vi "FilterSelectionParamSetting.vi"(8 "Error In":errorcluster, 10 "FiltersParam":T1={"Kernel"=[[1.0, 1.0, 1.0], [1.0, 1.0, 1.0], [1.0, 1.0, 1.0]], "Kernel Size"=0, "Filter Size X"=0, "Filter Size Y"=0, "Tolerance %"=0, "Divider"=0.0, "FilterFunction"=enum."Smoothing - Low Pass", "Sigma"=0.0, "LThres"=0.0, "HThresh"=0.0, "Windows Size"=0} {"Kernel Size" min=3 max=7 step=2}, 11 "FiltersParam":refnum<vi>) -> (0 "Error Out":errorcluster)   [LabVIEW 2019]
uses:
  Controls/FiltersParam_Type.ctl
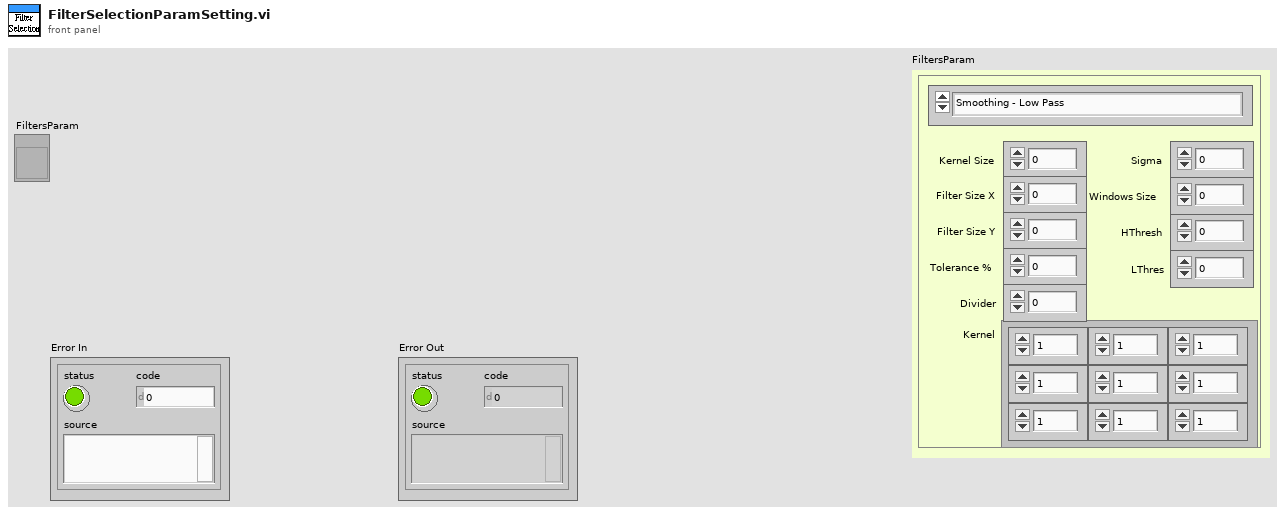
[diagram p1: front panel]
types:
  T1 = typedef "FiltersParam_Type.ctl" = cluster{"Kernel":sgl[][], "Kernel Size":i32, "Filter Size X":i32, "Filter Size Y":i32, "Tolerance %":i32, "Divider":sgl, "FilterFunction":enum16{"Smoothing - Low Pass", "Smoothing - Local Average", "Smoothing - Guassian", "Smoothing - Median", "------------------------------------", "Edge Detection - Laplacian", "Edge Detection - Diff", "Edge Detection - Prewitt", "Edge Detection - Sobel", "Edge Detection - Roberts", "Edge Detection - Canny", "Edge Detection - Gradient", "Edge Detection - Sigma", "----------------------------------------", "Convolution - Highlight Details", "Convolution - Custom"}, "Sigma":sgl, "LThres":sgl, "HThresh":sgl, "Windows Size":i32}
  T2 = enum16{"Smoothing - Low Pass", "Smoothing - Local Average", "Smoothing - Guassian", "Smoothing - Median", "------------------------------------", "Edge Detection - Laplacian", "Edge Detection - Diff", "Edge Detection - Prewitt", "Edge Detection - Sobel", "Edge Detection - Roberts", "Edge Detection - Canny", "Edge Detection - Gradient", "Edge Detection - Sigma", "----------------------------------------", "Convolution - Highlight Details", "Convolution - Custom"}
  T3 = enum8{"Enabled", "Disabled", "Disabled and Grayed Out"}
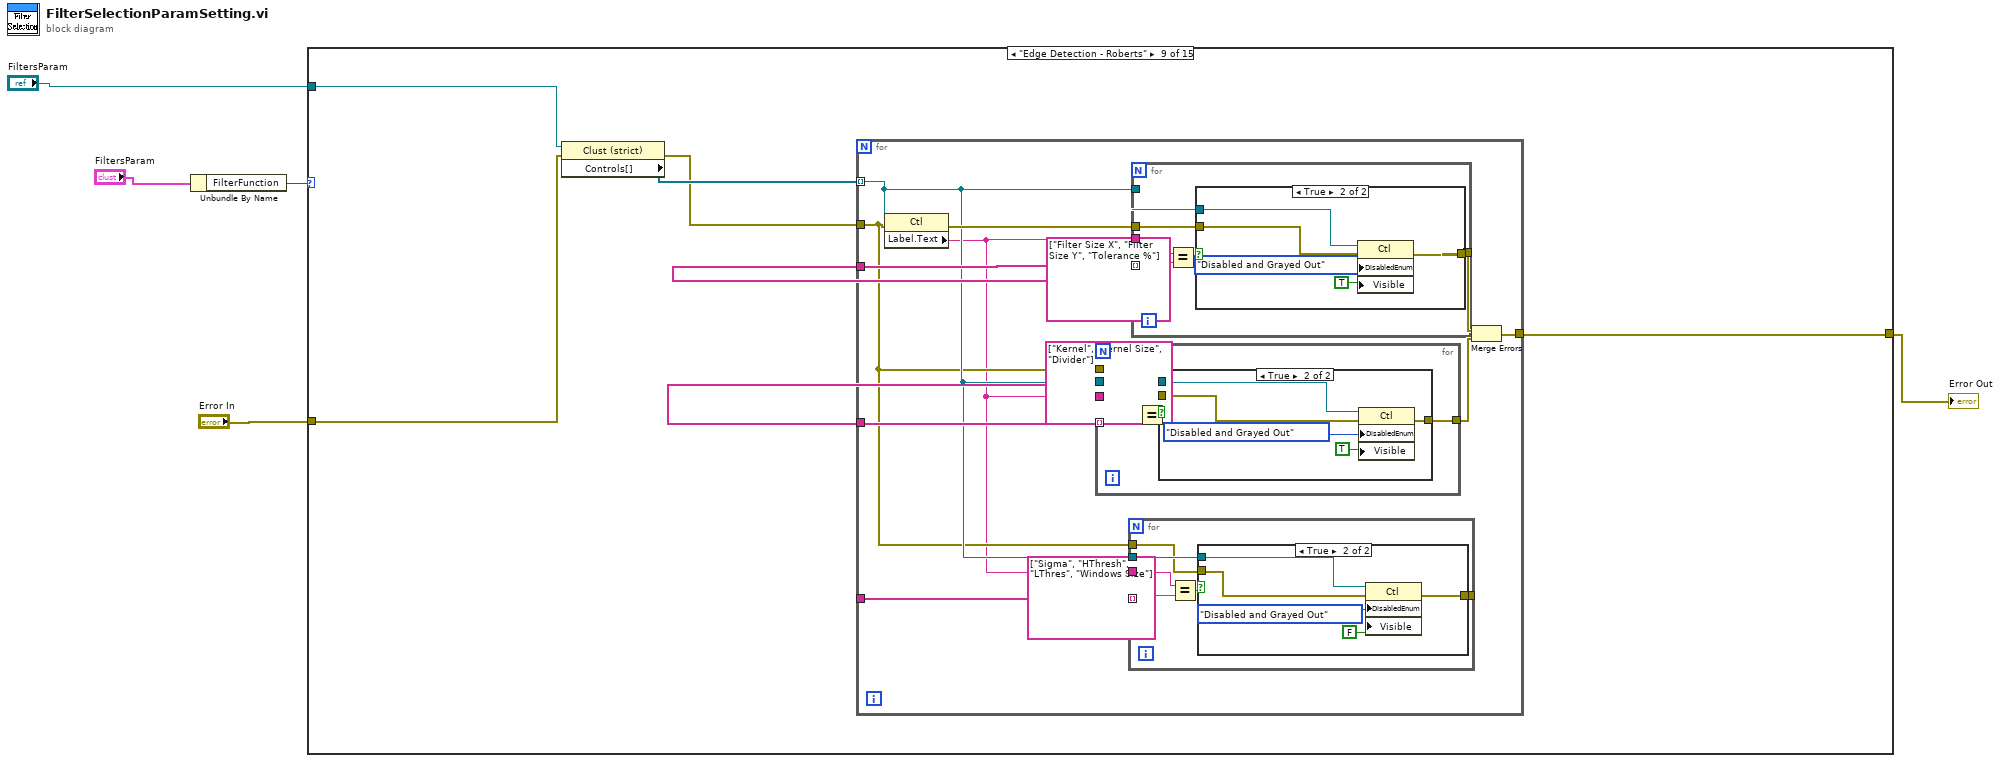
[diagram p0: block diagram]
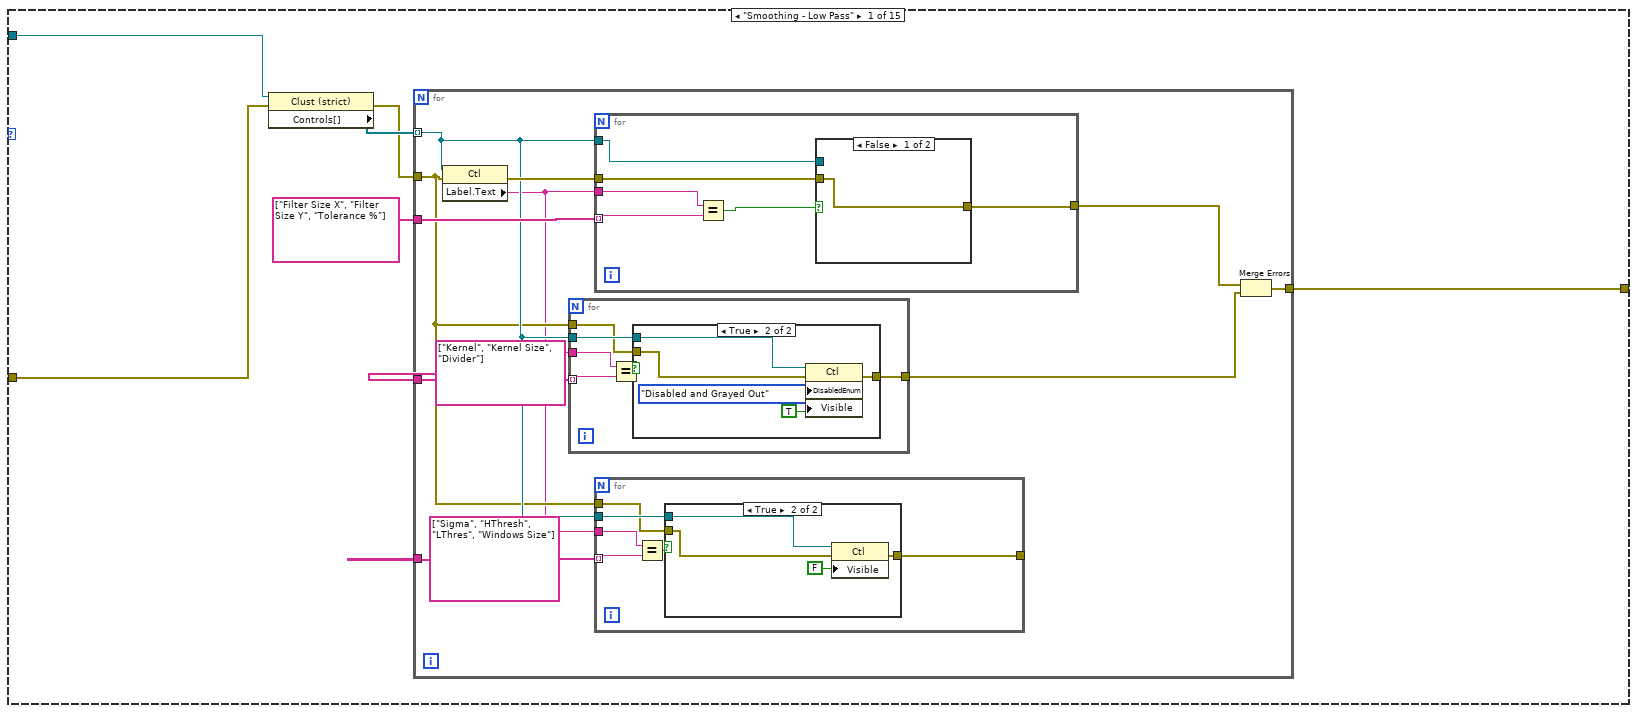
[diagram p2: hidden frame]
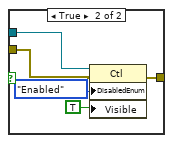
[diagram p5: hidden frame]
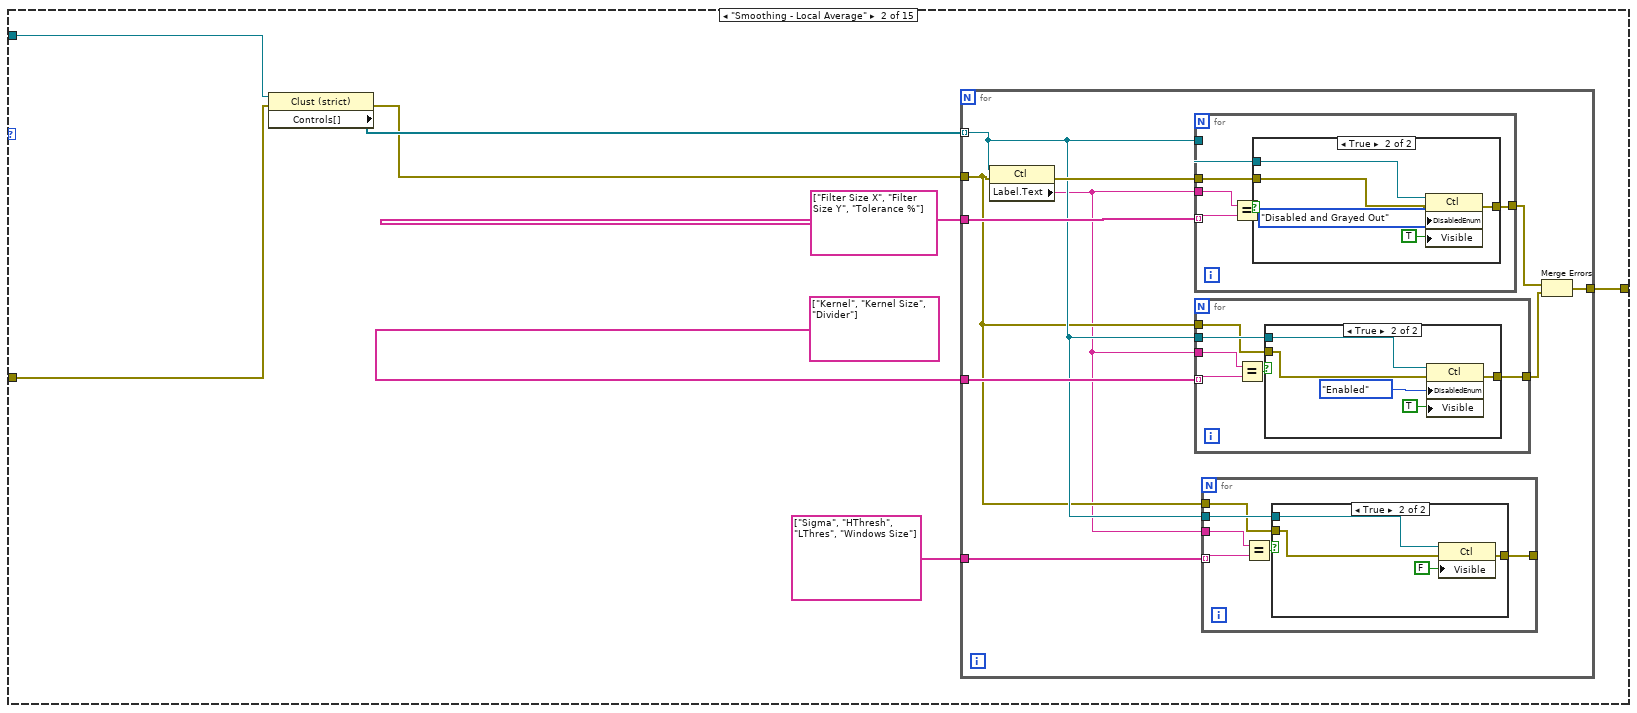
[diagram p6: hidden frame]
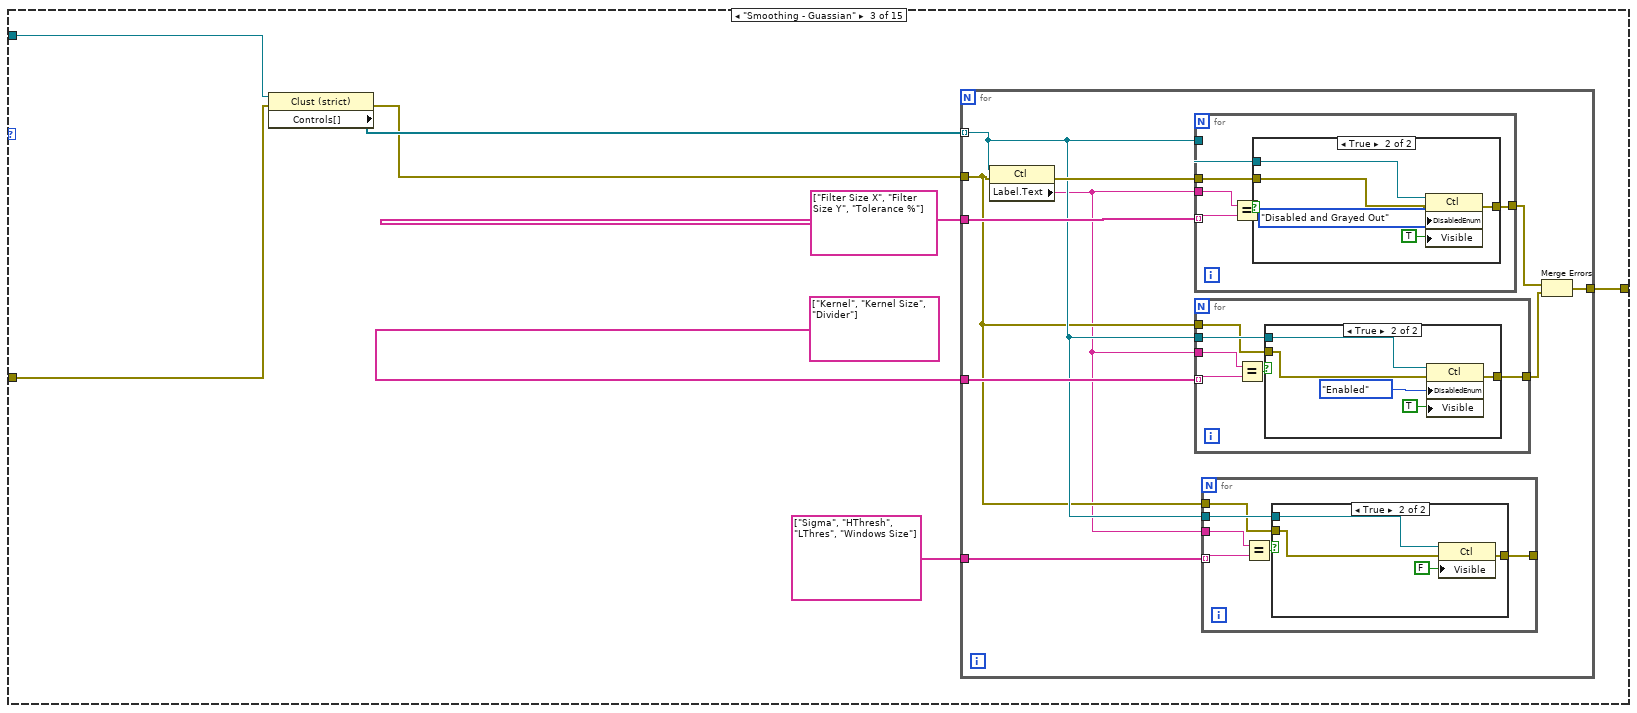
[diagram p10: hidden frame]
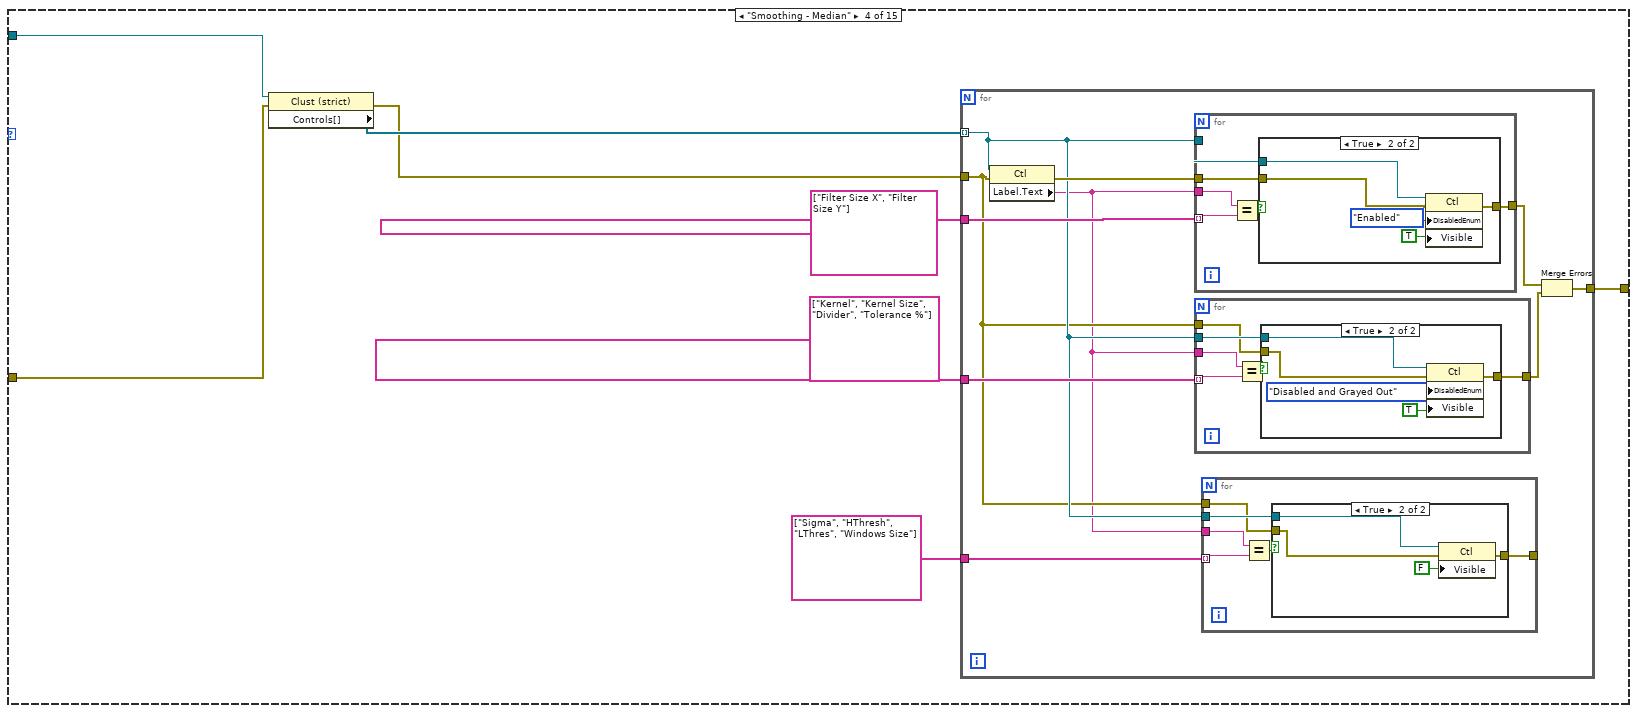
[diagram p14: hidden frame]
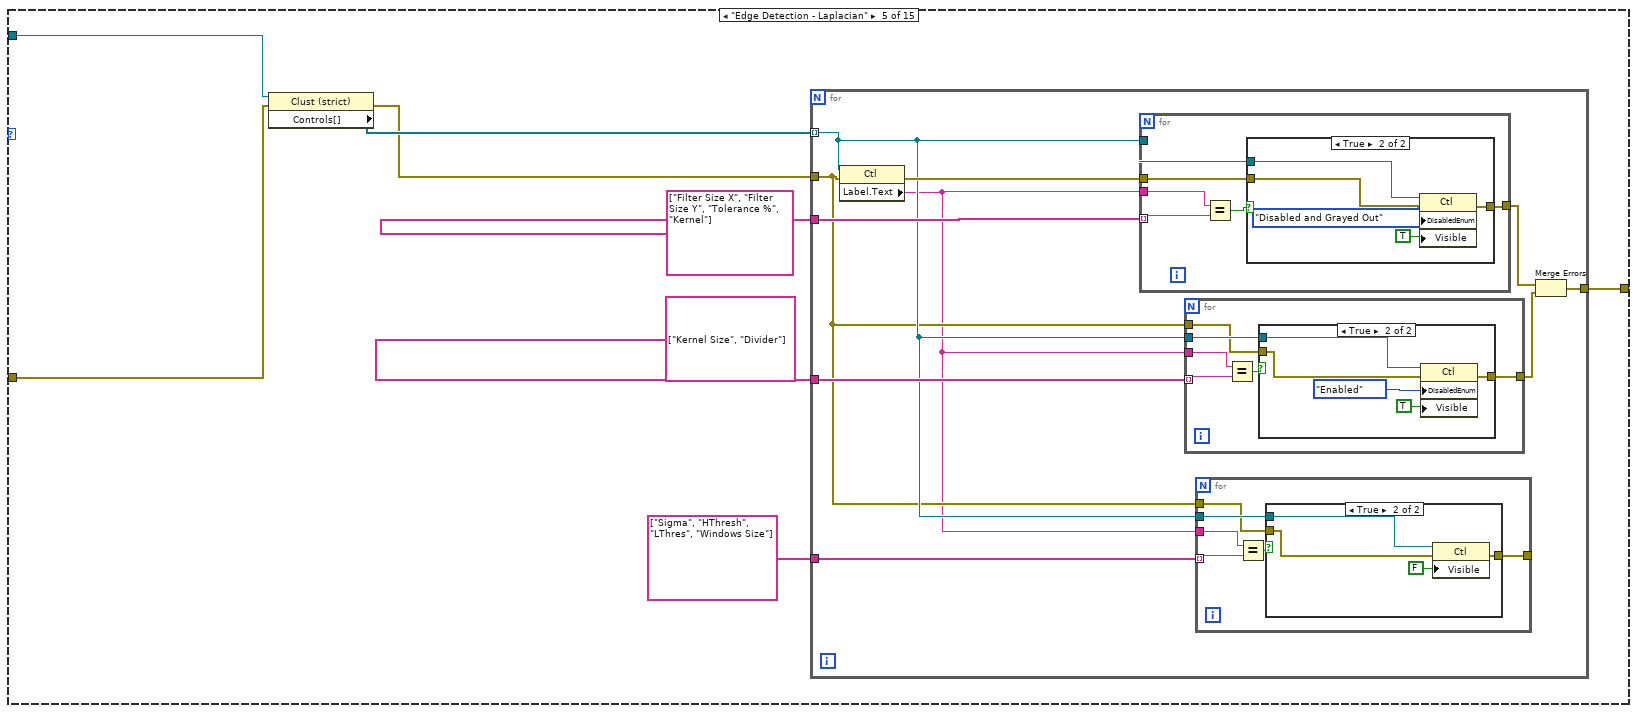
[diagram p18: hidden frame]
diagram:
  n1 = Unbundle By Name("FiltersParam") -> ("FilterFunction"=w4:T2)
  n2 = case shown="\"Edge Detection - Roberts\"" w4 {
    tunnel: "FiltersParam" -> [w13 w66 w119 w172 w225 w278 w331 w384 w438 w492 w546 w600 w654 _ _]
    tunnel: "Error In" -> [w9 w62 w115 w168 w221 w274 w327 w380 w434 w488 w542 w596 w650 w701 w702]
    tunnel: [w7 w60 w113 w166 w219 w272 w325 w378 w432 w486 w540 w594 w648 w701 w702] -> w3
    frame "Smoothing - Low Pass" {
      n3 = property class="Clust (strict)"(reference=w13, error in=w9) -> (error out=w8:errorcluster, "Controls[]"=w12:refnum<vi>[])  [unwired: 1 out]
      n4 = for {
        tunnel: w12 -> [w17] mode=indexing
        tunnel: string[] ["Filter Size X", "Filter Size Y", "Tolerance %"] -> [w23]
        tunnel: string[] ["Kernel", "Kernel Size", "Divider"] -> [w22]
        tunnel: w8 -> [w16]
        tunnel: [w18] -> w7
        tunnel: string[] ["Sigma", "HThresh", "LThres", "Windows Size"] -> [w15]
        n5 = property class="Ctl"(reference=w17, error in=w16) -> (error out=w21:errorcluster, "Label.Text"=w14:string)  [unwired: 1 out]
        n6 = for {
          tunnel: w14 -> [w40]
          tunnel: w22 -> [w39] mode=indexing
          tunnel: w17 -> [w37]
          tunnel: w16 -> [w36]
          tunnel: [w35] -> w19
          n7 = Equal?(x=w40, y=w39) -> (x = y?=w38:bool)
          n8 = case shown="True" w38 {
            tunnel: w37 -> [_ w46]
            tunnel: w36 -> [w41 w44]
            tunnel: [w41 w43] -> w35
            frame False {
            }
            frame True {
              n9 = property class="Ctl"(reference=w46, error in=w44, "DisabledEnum"=T3."Disabled and Grayed Out" ("Disabled"), "Visible"=TRUE) -> (error out=w43:errorcluster)  [unwired: 1 out]
            }
          }
        }
        n10 = for {
          tunnel: w14 -> [w52]
          tunnel: w23 -> [w51] mode=indexing
          tunnel: w17 -> [w49]
          tunnel: w21 -> [w48]
          tunnel: [w47] -> w20
          n11 = Equal?(x=w52, y=w51) -> (x = y?=w50:bool)
          n12 = case shown="False" w50 {
            tunnel: w49 -> [_ w58]
            tunnel: w48 -> [w53 w56]
            tunnel: [w53 w55] -> w47
            frame False {
            }
            frame True {
              n13 = property class="Ctl"(reference=w58, error in=w56, "DisabledEnum"=T3."Enabled" ("Disabled"), "Visible"=TRUE) -> (error out=w55:errorcluster)  [unwired: 1 out]
            }
          }
        }
        n14 = for {
          tunnel: w14 -> [w29]
          tunnel: w15 -> [w28] mode=indexing
          tunnel: w17 -> [w26]
          tunnel: w16 -> [w25]
          tunnel: [w24] -> _
          n15 = Equal?(x=w29, y=w28) -> (x = y?=w27:bool)
          n16 = case shown="True" w27 {
            tunnel: w26 -> [_ w34]
            tunnel: w25 -> [w30 w33]
            tunnel: [w30 w32] -> w24
            frame False {
            }
            frame True {
              n17 = property class="Ctl"(reference=w34, error in=w33, "Visible"=FALSE) -> (error out=w32:errorcluster)  [unwired: 1 out]
            }
          }
        }
        n18 = Merge Errors(w20, w19) -> (w18:errorcluster)
      }
    }
    frame "Smoothing - Local Average" {
      n19 = property class="Clust (strict)"(reference=w66, error in=w62) -> (error out=w61:errorcluster, "Controls[]"=w65:refnum<vi>[])  [unwired: 1 out]
      n20 = for {
        tunnel: w65 -> [w70] mode=indexing
        tunnel: string[] ["Filter Size X", "Filter Size Y", "Tolerance %"] -> [w76]
        tunnel: string[] ["Kernel", "Kernel Size", "Divider"] -> [w75]
        tunnel: w61 -> [w69]
        tunnel: [w71] -> w60
        tunnel: string[] ["Sigma", "HThresh", "LThres", "Windows Size"] -> [w68]
        n21 = property class="Ctl"(reference=w70, error in=w69) -> (error out=w74:errorcluster, "Label.Text"=w67:string)  [unwired: 1 out]
        n22 = for {
          tunnel: w67 -> [w105]
          tunnel: w76 -> [w104] mode=indexing
          tunnel: w70 -> [w102]
          tunnel: w74 -> [w101]
          tunnel: [w100] -> w73
          n23 = Equal?(x=w105, y=w104) -> (x = y?=w103:bool)
          n24 = case shown="True" w103 {
            tunnel: w102 -> [_ w111]
            tunnel: w101 -> [w106 w109]
            tunnel: [w106 w108] -> w100
            frame False {
            }
            frame True {
              n25 = property class="Ctl"(reference=w111, error in=w109, "DisabledEnum"=T3."Disabled and Grayed Out" ("Disabled"), "Visible"=TRUE) -> (error out=w108:errorcluster)  [unwired: 1 out]
            }
          }
        }
        n26 = for {
          tunnel: w67 -> [w93]
          tunnel: w75 -> [w92] mode=indexing
          tunnel: w70 -> [w90]
          tunnel: w69 -> [w89]
          tunnel: [w88] -> w72
          n27 = Equal?(x=w93, y=w92) -> (x = y?=w91:bool)
          n28 = case shown="True" w91 {
            tunnel: w90 -> [_ w99]
            tunnel: w89 -> [w94 w97]
            tunnel: [w94 w96] -> w88
            frame False {
            }
            frame True {
              n29 = property class="Ctl"(reference=w99, error in=w97, "DisabledEnum"=T3."Enabled" ("Disabled"), "Visible"=TRUE) -> (error out=w96:errorcluster)  [unwired: 1 out]
            }
          }
        }
        n30 = for {
          tunnel: w67 -> [w82]
          tunnel: w68 -> [w81] mode=indexing
          tunnel: w70 -> [w79]
          tunnel: w69 -> [w78]
          tunnel: [w77] -> _
          n31 = Equal?(x=w82, y=w81) -> (x = y?=w80:bool)
          n32 = case shown="True" w80 {
            tunnel: w79 -> [_ w87]
            tunnel: w78 -> [w83 w86]
            tunnel: [w83 w85] -> w77
            frame False {
            }
            frame True {
              n33 = property class="Ctl"(reference=w87, error in=w86, "Visible"=FALSE) -> (error out=w85:errorcluster)  [unwired: 1 out]
            }
          }
        }
        n34 = Merge Errors(w73, w72) -> (w71:errorcluster)
      }
    }
    frame "Smoothing - Guassian" {
      n35 = property class="Clust (strict)"(reference=w119, error in=w115) -> (error out=w114:errorcluster, "Controls[]"=w118:refnum<vi>[])  [unwired: 1 out]
      n36 = for {
        tunnel: w118 -> [w123] mode=indexing
        tunnel: string[] ["Filter Size X", "Filter Size Y", "Tolerance %"] -> [w129]
        tunnel: string[] ["Kernel", "Kernel Size", "Divider"] -> [w128]
        tunnel: w114 -> [w122]
        tunnel: [w124] -> w113
        tunnel: string[] ["Sigma", "HThresh", "LThres", "Windows Size"] -> [w121]
        n37 = property class="Ctl"(reference=w123, error in=w122) -> (error out=w127:errorcluster, "Label.Text"=w120:string)  [unwired: 1 out]
        n38 = for {
          tunnel: w120 -> [w158]
          tunnel: w129 -> [w157] mode=indexing
          tunnel: w123 -> [w155]
          tunnel: w127 -> [w154]
          tunnel: [w153] -> w126
          n39 = Equal?(x=w158, y=w157) -> (x = y?=w156:bool)
          n40 = case shown="True" w156 {
            tunnel: w155 -> [_ w164]
            tunnel: w154 -> [w159 w162]
            tunnel: [w159 w161] -> w153
            frame False {
            }
            frame True {
              n41 = property class="Ctl"(reference=w164, error in=w162, "DisabledEnum"=T3."Disabled and Grayed Out" ("Disabled"), "Visible"=TRUE) -> (error out=w161:errorcluster)  [unwired: 1 out]
            }
          }
        }
        n42 = for {
          tunnel: w120 -> [w146]
          tunnel: w128 -> [w145] mode=indexing
          tunnel: w123 -> [w143]
          tunnel: w122 -> [w142]
          tunnel: [w141] -> w125
          n43 = Equal?(x=w146, y=w145) -> (x = y?=w144:bool)
          n44 = case shown="True" w144 {
            tunnel: w143 -> [_ w152]
            tunnel: w142 -> [w147 w150]
            tunnel: [w147 w149] -> w141
            frame False {
            }
            frame True {
              n45 = property class="Ctl"(reference=w152, error in=w150, "DisabledEnum"=T3."Enabled" ("Disabled"), "Visible"=TRUE) -> (error out=w149:errorcluster)  [unwired: 1 out]
            }
          }
        }
        n46 = for {
          tunnel: w120 -> [w135]
          tunnel: w121 -> [w134] mode=indexing
          tunnel: w123 -> [w132]
          tunnel: w122 -> [w131]
          tunnel: [w130] -> _
          n47 = Equal?(x=w135, y=w134) -> (x = y?=w133:bool)
          n48 = case shown="True" w133 {
            tunnel: w132 -> [_ w140]
            tunnel: w131 -> [w136 w139]
            tunnel: [w136 w138] -> w130
            frame False {
            }
            frame True {
              n49 = property class="Ctl"(reference=w140, error in=w139, "Visible"=FALSE) -> (error out=w138:errorcluster)  [unwired: 1 out]
            }
          }
        }
        n50 = Merge Errors(w126, w125) -> (w124:errorcluster)
      }
    }
    frame "Smoothing - Median" {
      n51 = property class="Clust (strict)"(reference=w172, error in=w168) -> (error out=w167:errorcluster, "Controls[]"=w171:refnum<vi>[])  [unwired: 1 out]
      n52 = for {
        tunnel: w171 -> [w176] mode=indexing
        tunnel: string[] ["Filter Size X", "Filter Size Y"] -> [w182]
        tunnel: string[] ["Kernel", "Kernel Size", "Divider", "Tolerance %"] -> [w181]
        tunnel: w167 -> [w175]
        tunnel: [w177] -> w166
        tunnel: string[] ["Sigma", "HThresh", "LThres", "Windows Size"] -> [w174]
        n53 = property class="Ctl"(reference=w176, error in=w175) -> (error out=w180:errorcluster, "Label.Text"=w173:string)  [unwired: 1 out]
        n54 = for {
          tunnel: w173 -> [w211]
          tunnel: w182 -> [w210] mode=indexing
          tunnel: w176 -> [w208]
          tunnel: w180 -> [w207]
          tunnel: [w206] -> w179
          n55 = Equal?(x=w211, y=w210) -> (x = y?=w209:bool)
          n56 = case shown="True" w209 {
            tunnel: w208 -> [_ w217]
            tunnel: w207 -> [w212 w215]
            tunnel: [w212 w214] -> w206
            frame False {
            }
            frame True {
              n57 = property class="Ctl"(reference=w217, error in=w215, "DisabledEnum"=T3."Enabled" ("Disabled"), "Visible"=TRUE) -> (error out=w214:errorcluster)  [unwired: 1 out]
            }
          }
        }
        n58 = for {
          tunnel: w173 -> [w199]
          tunnel: w181 -> [w198] mode=indexing
          tunnel: w176 -> [w196]
          tunnel: w175 -> [w195]
          tunnel: [w194] -> w178
          n59 = Equal?(x=w199, y=w198) -> (x = y?=w197:bool)
          n60 = case shown="True" w197 {
            tunnel: w196 -> [_ w205]
            tunnel: w195 -> [w200 w203]
            tunnel: [w200 w202] -> w194
            frame False {
            }
            frame True {
              n61 = property class="Ctl"(reference=w205, error in=w203, "DisabledEnum"=T3."Disabled and Grayed Out" ("Disabled"), "Visible"=TRUE) -> (error out=w202:errorcluster)  [unwired: 1 out]
            }
          }
        }
        n62 = for {
          tunnel: w173 -> [w188]
          tunnel: w174 -> [w187] mode=indexing
          tunnel: w176 -> [w185]
          tunnel: w175 -> [w184]
          tunnel: [w183] -> _
          n63 = Equal?(x=w188, y=w187) -> (x = y?=w186:bool)
          n64 = case shown="True" w186 {
            tunnel: w185 -> [_ w193]
            tunnel: w184 -> [w189 w192]
            tunnel: [w189 w191] -> w183
            frame False {
            }
            frame True {
              n65 = property class="Ctl"(reference=w193, error in=w192, "Visible"=FALSE) -> (error out=w191:errorcluster)  [unwired: 1 out]
            }
          }
        }
        n66 = Merge Errors(w179, w178) -> (w177:errorcluster)
      }
    }
    frame "Edge Detection - Laplacian" {
      n67 = property class="Clust (strict)"(reference=w225, error in=w221) -> (error out=w220:errorcluster, "Controls[]"=w224:refnum<vi>[])  [unwired: 1 out]
      n68 = for {
        tunnel: w224 -> [w229] mode=indexing
        tunnel: string[] ["Filter Size X", "Filter Size Y", "Tolerance %", "Kernel"] -> [w235]
        tunnel: string[] ["Kernel Size", "Divider"] -> [w234]
        tunnel: w220 -> [w228]
        tunnel: [w230] -> w219
        tunnel: string[] ["Sigma", "HThresh", "LThres", "Windows Size"] -> [w227]
        n69 = property class="Ctl"(reference=w229, error in=w228) -> (error out=w233:errorcluster, "Label.Text"=w226:string)  [unwired: 1 out]
        n70 = for {
          tunnel: w226 -> [w264]
          tunnel: w235 -> [w263] mode=indexing
          tunnel: w229 -> [w261]
          tunnel: w233 -> [w260]
          tunnel: [w259] -> w232
          n71 = Equal?(x=w264, y=w263) -> (x = y?=w262:bool)
          n72 = case shown="True" w262 {
            tunnel: w261 -> [_ w270]
            tunnel: w260 -> [w265 w268]
            tunnel: [w265 w267] -> w259
            frame False {
            }
            frame True {
              n73 = property class="Ctl"(reference=w270, error in=w268, "DisabledEnum"=T3."Disabled and Grayed Out" ("Disabled"), "Visible"=TRUE) -> (error out=w267:errorcluster)  [unwired: 1 out]
            }
          }
        }
        n74 = for {
          tunnel: w226 -> [w252]
          tunnel: w234 -> [w251] mode=indexing
          tunnel: w229 -> [w249]
          tunnel: w228 -> [w248]
          tunnel: [w247] -> w231
          n75 = Equal?(x=w252, y=w251) -> (x = y?=w250:bool)
          n76 = case shown="True" w250 {
            tunnel: w249 -> [_ w258]
            tunnel: w248 -> [w253 w256]
            tunnel: [w253 w255] -> w247
            frame False {
            }
            frame True {
              n77 = property class="Ctl"(reference=w258, error in=w256, "DisabledEnum"=T3."Enabled" ("Disabled"), "Visible"=TRUE) -> (error out=w255:errorcluster)  [unwired: 1 out]
            }
          }
        }
        n78 = for {
          tunnel: w226 -> [w241]
          tunnel: w227 -> [w240] mode=indexing
          tunnel: w229 -> [w238]
          tunnel: w228 -> [w237]
          tunnel: [w236] -> _
          n79 = Equal?(x=w241, y=w240) -> (x = y?=w239:bool)
          n80 = case shown="True" w239 {
            tunnel: w238 -> [_ w246]
            tunnel: w237 -> [w242 w245]
            tunnel: [w242 w244] -> w236
            frame False {
            }
            frame True {
              n81 = property class="Ctl"(reference=w246, error in=w245, "Visible"=FALSE) -> (error out=w244:errorcluster)  [unwired: 1 out]
            }
          }
        }
        n82 = Merge Errors(w232, w231) -> (w230:errorcluster)
      }
    }
    frame "Edge Detection - Diff" {
      n83 = property class="Clust (strict)"(reference=w278, error in=w274) -> (error out=w273:errorcluster, "Controls[]"=w277:refnum<vi>[])  [unwired: 1 out]
      n84 = for {
        tunnel: w277 -> [w282] mode=indexing
        tunnel: string[] ["Filter Size X", "Filter Size Y", "Tolerance %"] -> [w288]
        tunnel: string[] ["Kernel", "Kernel Size", "Divider"] -> [w287]
        tunnel: w273 -> [w281]
        tunnel: [w283] -> w272
        tunnel: string[] ["Sigma", "HThresh", "LThres", "Windows Size"] -> [w280]
        n85 = property class="Ctl"(reference=w282, error in=w281) -> (error out=w286:errorcluster, "Label.Text"=w279:string)  [unwired: 1 out]
        n86 = for {
          tunnel: w279 -> [w317]
          tunnel: w288 -> [w316] mode=indexing
          tunnel: w282 -> [w314]
          tunnel: w286 -> [w313]
          tunnel: [w312] -> w285
          n87 = Equal?(x=w317, y=w316) -> (x = y?=w315:bool)
          n88 = case shown="True" w315 {
            tunnel: w314 -> [_ w323]
            tunnel: w313 -> [w318 w321]
            tunnel: [w318 w320] -> w312
            frame False {
            }
            frame True {
              n89 = property class="Ctl"(reference=w323, error in=w321, "DisabledEnum"=T3."Disabled and Grayed Out" ("Disabled"), "Visible"=TRUE) -> (error out=w320:errorcluster)  [unwired: 1 out]
            }
          }
        }
        n90 = for {
          tunnel: w279 -> [w305]
          tunnel: w287 -> [w304] mode=indexing
          tunnel: w282 -> [w302]
          tunnel: w281 -> [w301]
          tunnel: [w300] -> w284
          n91 = Equal?(x=w305, y=w304) -> (x = y?=w303:bool)
          n92 = case shown="True" w303 {
            tunnel: w302 -> [_ w311]
            tunnel: w301 -> [w306 w309]
            tunnel: [w306 w308] -> w300
            frame False {
            }
            frame True {
              n93 = property class="Ctl"(reference=w311, error in=w309, "DisabledEnum"=T3."Disabled and Grayed Out" ("Disabled"), "Visible"=TRUE) -> (error out=w308:errorcluster)  [unwired: 1 out]
            }
          }
        }
        n94 = for {
          tunnel: w279 -> [w294]
          tunnel: w280 -> [w293] mode=indexing
          tunnel: w282 -> [w291]
          tunnel: w281 -> [w290]
          tunnel: [w289] -> _
          n95 = Equal?(x=w294, y=w293) -> (x = y?=w292:bool)
          n96 = case shown="True" w292 {
            tunnel: w291 -> [_ w299]
            tunnel: w290 -> [w295 w298]
            tunnel: [w295 w297] -> w289
            frame False {
            }
            frame True {
              n97 = property class="Ctl"(reference=w299, error in=w298, "Visible"=FALSE) -> (error out=w297:errorcluster)  [unwired: 1 out]
            }
          }
        }
        n98 = Merge Errors(w285, w284) -> (w283:errorcluster)
      }
    }
    frame "Edge Detection - Prewitt" {
      n99 = property class="Clust (strict)"(reference=w331, error in=w327) -> (error out=w326:errorcluster, "Controls[]"=w330:refnum<vi>[])  [unwired: 1 out]
      n100 = for {
        tunnel: w330 -> [w335] mode=indexing
        tunnel: string[] ["Filter Size X", "Filter Size Y", "Tolerance %"] -> [w341]
        tunnel: string[] ["Kernel", "Kernel Size", "Divider"] -> [w340]
        tunnel: w326 -> [w334]
        tunnel: [w336] -> w325
        tunnel: string[] ["Sigma", "HThresh", "LThres", "Windows Size"] -> [w333]
        n101 = property class="Ctl"(reference=w335, error in=w334) -> (error out=w339:errorcluster, "Label.Text"=w332:string)  [unwired: 1 out]
        n102 = for {
          tunnel: w332 -> [w358]
          tunnel: w340 -> [w357] mode=indexing
          tunnel: w335 -> [w355]
          tunnel: w334 -> [w354]
          tunnel: [w353] -> w337
          n103 = Equal?(x=w358, y=w357) -> (x = y?=w356:bool)
          n104 = case shown="True" w356 {
            tunnel: w355 -> [_ w364]
            tunnel: w354 -> [w359 w362]
            tunnel: [w359 w361] -> w353
            frame False {
            }
            frame True {
              n105 = property class="Ctl"(reference=w364, error in=w362, "DisabledEnum"=T3."Disabled and Grayed Out" ("Disabled"), "Visible"=TRUE) -> (error out=w361:errorcluster)  [unwired: 1 out]
            }
          }
        }
        n106 = for {
          tunnel: w332 -> [w370]
          tunnel: w341 -> [w369] mode=indexing
          tunnel: w335 -> [w367]
          tunnel: w339 -> [w366]
          tunnel: [w365] -> w338
          n107 = Equal?(x=w370, y=w369) -> (x = y?=w368:bool)
          n108 = case shown="True" w368 {
            tunnel: w367 -> [_ w376]
            tunnel: w366 -> [w371 w374]
            tunnel: [w371 w373] -> w365
            frame False {
            }
            frame True {
              n109 = property class="Ctl"(reference=w376, error in=w374, "DisabledEnum"=T3."Disabled and Grayed Out" ("Disabled"), "Visible"=TRUE) -> (error out=w373:errorcluster)  [unwired: 1 out]
            }
          }
        }
        n110 = for {
          tunnel: w332 -> [w347]
          tunnel: w333 -> [w346] mode=indexing
          tunnel: w335 -> [w344]
          tunnel: w334 -> [w343]
          tunnel: [w342] -> _
          n111 = Equal?(x=w347, y=w346) -> (x = y?=w345:bool)
          n112 = case shown="True" w345 {
            tunnel: w344 -> [_ w352]
            tunnel: w343 -> [w348 w351]
            tunnel: [w348 w350] -> w342
            frame False {
            }
            frame True {
              n113 = property class="Ctl"(reference=w352, error in=w351, "Visible"=FALSE) -> (error out=w350:errorcluster)  [unwired: 1 out]
            }
          }
        }
        n114 = Merge Errors(w338, w337) -> (w336:errorcluster)
      }
    }
    frame "Edge Detection - Sobel" {
      n115 = property class="Clust (strict)"(reference=w384, error in=w380) -> (error out=w379:errorcluster, "Controls[]"=w383:refnum<vi>[])  [unwired: 1 out]
      n116 = for {
        tunnel: w383 -> [w388] mode=indexing
        tunnel: string[] ["Filter Size X", "Filter Size Y", "Tolerance %"] -> [w394]
        tunnel: string[] ["Kernel", "Kernel Size", "Divider"] -> [w393]
        tunnel: w379 -> [w387]
        tunnel: [w389] -> w378
        tunnel: string[] ["Sigma", "HThresh", "LThres", "Windows Size"] -> [w386]
        n117 = property class="Ctl"(reference=w388, error in=w387) -> (error out=w392:errorcluster, "Label.Text"=w385:string)  [unwired: 1 out]
        n118 = for {
          tunnel: w385 -> [w412]
          tunnel: w393 -> [w411] mode=indexing
          tunnel: w388 -> [w409]
          tunnel: w387 -> [w408]
          tunnel: [w407] -> w390
          n119 = Equal?(x=w412, y=w411) -> (x = y?=w410:bool)
          n120 = case shown="True" w410 {
            tunnel: w409 -> [_ w418]
            tunnel: w408 -> [w413 w416]
            tunnel: [w413 w415] -> w407
            frame False {
            }
            frame True {
              n121 = property class="Ctl"(reference=w418, error in=w416, "DisabledEnum"=T3."Disabled and Grayed Out" ("Disabled"), "Visible"=TRUE) -> (error out=w415:errorcluster)  [unwired: 1 out]
            }
          }
        }
        n122 = for {
          tunnel: w385 -> [w424]
          tunnel: w394 -> [w423] mode=indexing
          tunnel: w388 -> [w421]
          tunnel: w392 -> [w420]
          tunnel: [w419] -> w391
          n123 = Equal?(x=w424, y=w423) -> (x = y?=w422:bool)
          n124 = case shown="True" w422 {
            tunnel: w421 -> [_ w430]
            tunnel: w420 -> [w425 w428]
            tunnel: [w425 w427] -> w419
            frame False {
            }
            frame True {
              n125 = property class="Ctl"(reference=w430, error in=w428, "DisabledEnum"=T3."Disabled and Grayed Out" ("Disabled"), "Visible"=TRUE) -> (error out=w427:errorcluster)  [unwired: 1 out]
            }
          }
        }
        n126 = for {
          tunnel: w385 -> [w400]
          tunnel: w386 -> [w399] mode=indexing
          tunnel: w388 -> [w397]
          tunnel: w387 -> [w396]
          tunnel: [w395] -> _
          n127 = Equal?(x=w400, y=w399) -> (x = y?=w398:bool)
          n128 = case shown="True" w398 {
            tunnel: w397 -> [_ w406]
            tunnel: w396 -> [w401 w404]
            tunnel: [w401 w403] -> w395
            frame False {
            }
            frame True {
              n129 = property class="Ctl"(reference=w406, error in=w404, "DisabledEnum"=T3."Disabled and Grayed Out" ("Disabled"), "Visible"=FALSE) -> (error out=w403:errorcluster)  [unwired: 1 out]
            }
          }
        }
        n130 = Merge Errors(w391, w390) -> (w389:errorcluster)
      }
    }
    frame "Edge Detection - Roberts" {
      n131 = property class="Clust (strict)"(reference=w438, error in=w434) -> (error out=w433:errorcluster, "Controls[]"=w437:refnum<vi>[])  [unwired: 1 out]
      n132 = for {
        tunnel: w437 -> [w442] mode=indexing
        tunnel: string[] ["Filter Size X", "Filter Size Y", "Tolerance %"] -> [w448]
        tunnel: string[] ["Kernel", "Kernel Size", "Divider"] -> [w447]
        tunnel: w433 -> [w441]
        tunnel: [w443] -> w432
        tunnel: string[] ["Sigma", "HThresh", "LThres", "Windows Size"] -> [w440]
        n133 = property class="Ctl"(reference=w442, error in=w441) -> (error out=w446:errorcluster, "Label.Text"=w439:string)  [unwired: 1 out]
        n134 = for {
          tunnel: w439 -> [w466]
          tunnel: w447 -> [w465] mode=indexing
          tunnel: w442 -> [w463]
          tunnel: w441 -> [w462]
          tunnel: [w461] -> w444
          n135 = Equal?(x=w466, y=w465) -> (x = y?=w464:bool)
          n136 = case shown="True" w464 {
            tunnel: w463 -> [_ w472]
            tunnel: w462 -> [w467 w470]
            tunnel: [w467 w469] -> w461
            frame False {
            }
            frame True {
              n137 = property class="Ctl"(reference=w472, error in=w470, "DisabledEnum"=T3."Disabled and Grayed Out" ("Disabled"), "Visible"=TRUE) -> (error out=w469:errorcluster)  [unwired: 1 out]
            }
          }
        }
        n138 = for {
          tunnel: w439 -> [w454]
          tunnel: w440 -> [w453] mode=indexing
          tunnel: w442 -> [w451]
          tunnel: w441 -> [w450]
          tunnel: [w449] -> _
          n139 = Equal?(x=w454, y=w453) -> (x = y?=w452:bool)
          n140 = case shown="True" w452 {
            tunnel: w451 -> [_ w460]
            tunnel: w450 -> [w455 w458]
            tunnel: [w455 w457] -> w449
            frame False {
            }
            frame True {
              n141 = property class="Ctl"(reference=w460, error in=w458, "DisabledEnum"=T3."Disabled and Grayed Out" ("Disabled"), "Visible"=FALSE) -> (error out=w457:errorcluster)  [unwired: 1 out]
            }
          }
        }
        n142 = for {
          tunnel: w439 -> [w478]
          tunnel: w448 -> [w477] mode=indexing
          tunnel: w442 -> [w475]
          tunnel: w446 -> [w474]
          tunnel: [w473] -> w445
          n143 = Equal?(x=w478, y=w477) -> (x = y?=w476:bool)
          n144 = case shown="True" w476 {
            tunnel: w475 -> [_ w484]
            tunnel: w474 -> [w479 w482]
            tunnel: [w479 w481] -> w473
            frame False {
            }
            frame True {
              n145 = property class="Ctl"(reference=w484, error in=w482, "DisabledEnum"=T3."Disabled and Grayed Out" ("Disabled"), "Visible"=TRUE) -> (error out=w481:errorcluster)  [unwired: 1 out]
            }
          }
        }
        n146 = Merge Errors(w445, w444) -> (w443:errorcluster)
      }
    }
    frame "Edge Detection - Gradient" {
      n147 = property class="Clust (strict)"(reference=w492, error in=w488) -> (error out=w487:errorcluster, "Controls[]"=w491:refnum<vi>[])  [unwired: 1 out]
      n148 = for {
        tunnel: w491 -> [w496] mode=indexing
        tunnel: string[] ["Filter Size X", "Filter Size Y", "Tolerance %"] -> [w502]
        tunnel: string[] ["Kernel", "Kernel Size", "Divider"] -> [w501]
        tunnel: w487 -> [w495]
        tunnel: [w497] -> w486
        tunnel: string[] ["Sigma", "HThresh", "LThres", "Windows Size"] -> [w494]
        n149 = property class="Ctl"(reference=w496, error in=w495) -> (error out=w500:errorcluster, "Label.Text"=w493:string)  [unwired: 1 out]
        n150 = for {
          tunnel: w493 -> [w520]
          tunnel: w501 -> [w519] mode=indexing
          tunnel: w496 -> [w517]
          tunnel: w495 -> [w516]
          tunnel: [w515] -> w498
          n151 = Equal?(x=w520, y=w519) -> (x = y?=w518:bool)
          n152 = case shown="True" w518 {
            tunnel: w517 -> [_ w526]
            tunnel: w516 -> [w521 w524]
            tunnel: [w521 w523] -> w515
            frame False {
            }
            frame True {
              n153 = property class="Ctl"(reference=w526, error in=w524, "DisabledEnum"=T3."Disabled and Grayed Out" ("Disabled"), "Visible"=TRUE) -> (error out=w523:errorcluster)  [unwired: 1 out]
            }
          }
        }
        n154 = for {
          tunnel: w493 -> [w508]
          tunnel: w494 -> [w507] mode=indexing
          tunnel: w496 -> [w505]
          tunnel: w495 -> [w504]
          tunnel: [w503] -> _
          n155 = Equal?(x=w508, y=w507) -> (x = y?=w506:bool)
          n156 = case shown="True" w506 {
            tunnel: w505 -> [_ w514]
            tunnel: w504 -> [w509 w512]
            tunnel: [w509 w511] -> w503
            frame False {
            }
            frame True {
              n157 = property class="Ctl"(reference=w514, error in=w512, "DisabledEnum"=T3."Disabled and Grayed Out" ("Disabled"), "Visible"=FALSE) -> (error out=w511:errorcluster)  [unwired: 1 out]
            }
          }
        }
        n158 = for {
          tunnel: w493 -> [w532]
          tunnel: w502 -> [w531] mode=indexing
          tunnel: w496 -> [w529]
          tunnel: w500 -> [w528]
          tunnel: [w527] -> w499
          n159 = Equal?(x=w532, y=w531) -> (x = y?=w530:bool)
          n160 = case shown="True" w530 {
            tunnel: w529 -> [_ w538]
            tunnel: w528 -> [w533 w536]
            tunnel: [w533 w535] -> w527
            frame False {
            }
            frame True {
              n161 = property class="Ctl"(reference=w538, error in=w536, "DisabledEnum"=T3."Disabled and Grayed Out" ("Disabled"), "Visible"=TRUE) -> (error out=w535:errorcluster)  [unwired: 1 out]
            }
          }
        }
        n162 = Merge Errors(w499, w498) -> (w497:errorcluster)
      }
    }
    frame "Edge Detection - Sigma" {
      n163 = property class="Clust (strict)"(reference=w546, error in=w542) -> (error out=w541:errorcluster, "Controls[]"=w545:refnum<vi>[])  [unwired: 1 out]
      n164 = for {
        tunnel: w545 -> [w550] mode=indexing
        tunnel: string[] ["Filter Size X", "Filter Size Y", "Tolerance %"] -> [w556]
        tunnel: string[] ["Kernel", "Kernel Size", "Divider"] -> [w555]
        tunnel: w541 -> [w549]
        tunnel: [w551] -> w540
        tunnel: string[] ["Sigma", "HThresh", "LThres", "Windows Size"] -> [w548]
        n165 = property class="Ctl"(reference=w550, error in=w549) -> (error out=w554:errorcluster, "Label.Text"=w547:string)  [unwired: 1 out]
        n166 = for {
          tunnel: w547 -> [w574]
          tunnel: w555 -> [w573] mode=indexing
          tunnel: w550 -> [w571]
          tunnel: w549 -> [w570]
          tunnel: [w569] -> w552
          n167 = Equal?(x=w574, y=w573) -> (x = y?=w572:bool)
          n168 = case shown="True" w572 {
            tunnel: w571 -> [_ w580]
            tunnel: w570 -> [w575 w578]
            tunnel: [w575 w577] -> w569
            frame False {
            }
            frame True {
              n169 = property class="Ctl"(reference=w580, error in=w578, "DisabledEnum"=T3."Disabled and Grayed Out" ("Disabled"), "Visible"=TRUE) -> (error out=w577:errorcluster)  [unwired: 1 out]
            }
          }
        }
        n170 = for {
          tunnel: w547 -> [w586]
          tunnel: w556 -> [w585] mode=indexing
          tunnel: w550 -> [w583]
          tunnel: w554 -> [w582]
          tunnel: [w581] -> w553
          n171 = Equal?(x=w586, y=w585) -> (x = y?=w584:bool)
          n172 = case shown="True" w584 {
            tunnel: w583 -> [_ w592]
            tunnel: w582 -> [w587 w590]
            tunnel: [w587 w589] -> w581
            frame False {
            }
            frame True {
              n173 = property class="Ctl"(reference=w592, error in=w590, "DisabledEnum"=T3."Disabled and Grayed Out" ("Disabled"), "Visible"=TRUE) -> (error out=w589:errorcluster)  [unwired: 1 out]
            }
          }
        }
        n174 = for {
          tunnel: w547 -> [w562]
          tunnel: w548 -> [w561] mode=indexing
          tunnel: w550 -> [w559]
          tunnel: w549 -> [w558]
          tunnel: [w557] -> _
          n175 = Equal?(x=w562, y=w561) -> (x = y?=w560:bool)
          n176 = case shown="True" w560 {
            tunnel: w559 -> [_ w568]
            tunnel: w558 -> [w563 w566]
            tunnel: [w563 w565] -> w557
            frame False {
            }
            frame True {
              n177 = property class="Ctl"(reference=w568, error in=w566, "DisabledEnum"=T3."Disabled and Grayed Out" ("Disabled"), "Visible"=FALSE) -> (error out=w565:errorcluster)  [unwired: 1 out]
            }
          }
        }
        n178 = Merge Errors(w553, w552) -> (w551:errorcluster)
      }
    }
    frame "Convolution - Highlight Details" {
      n179 = property class="Clust (strict)"(reference=w600, error in=w596) -> (error out=w595:errorcluster, "Controls[]"=w599:refnum<vi>[])  [unwired: 1 out]
      n180 = for {
        tunnel: w599 -> [w604] mode=indexing
        tunnel: string[] ["Filter Size X", "Filter Size Y", "Tolerance %"] -> [w610]
        tunnel: string[] ["Kernel", "Kernel Size", "Divider"] -> [w609]
        tunnel: w595 -> [w603]
        tunnel: [w605] -> w594
        tunnel: string[] ["Sigma", "HThresh", "LThres", "Windows Size"] -> [w602]
        n181 = property class="Ctl"(reference=w604, error in=w603) -> (error out=w608:errorcluster, "Label.Text"=w601:string)  [unwired: 1 out]
        n182 = for {
          tunnel: w601 -> [w628]
          tunnel: w609 -> [w627] mode=indexing
          tunnel: w604 -> [w625]
          tunnel: w603 -> [w624]
          tunnel: [w623] -> w606
          n183 = Equal?(x=w628, y=w627) -> (x = y?=w626:bool)
          n184 = case shown="True" w626 {
            tunnel: w625 -> [_ w634]
            tunnel: w624 -> [w629 w632]
            tunnel: [w629 w631] -> w623
            frame False {
            }
            frame True {
              n185 = property class="Ctl"(reference=w634, error in=w632, "DisabledEnum"=T3."Enabled" ("Disabled"), "Visible"=TRUE) -> (error out=w631:errorcluster)  [unwired: 1 out]
            }
          }
        }
        n186 = for {
          tunnel: w601 -> [w616]
          tunnel: w602 -> [w615] mode=indexing
          tunnel: w604 -> [w613]
          tunnel: w603 -> [w612]
          tunnel: [w611] -> _
          n187 = Equal?(x=w616, y=w615) -> (x = y?=w614:bool)
          n188 = case shown="True" w614 {
            tunnel: w613 -> [_ w622]
            tunnel: w612 -> [w617 w620]
            tunnel: [w617 w619] -> w611
            frame False {
            }
            frame True {
              n189 = property class="Ctl"(reference=w622, error in=w620, "DisabledEnum"=T3."Disabled and Grayed Out" ("Disabled"), "Visible"=FALSE) -> (error out=w619:errorcluster)  [unwired: 1 out]
            }
          }
        }
        n190 = for {
          tunnel: w601 -> [w640]
          tunnel: w610 -> [w639] mode=indexing
          tunnel: w604 -> [w637]
          tunnel: w608 -> [w636]
          tunnel: [w635] -> w607
          n191 = Equal?(x=w640, y=w639) -> (x = y?=w638:bool)
          n192 = case shown="True" w638 {
            tunnel: w637 -> [_ w646]
            tunnel: w636 -> [w641 w644]
            tunnel: [w641 w643] -> w635
            frame False {
            }
            frame True {
              n193 = property class="Ctl"(reference=w646, error in=w644, "DisabledEnum"=T3."Disabled and Grayed Out" ("Disabled"), "Visible"=TRUE) -> (error out=w643:errorcluster)  [unwired: 1 out]
            }
          }
        }
        n194 = Merge Errors(w607, w606) -> (w605:errorcluster)
      }
    }
    frame "Edge Detection - Canny" {
      n195 = property class="Clust (strict)"(reference=w654, error in=w650) -> (error out=w649:errorcluster, "Controls[]"=w653:refnum<vi>[])  [unwired: 1 out]
      n196 = for {
        tunnel: w653 -> [w658] mode=indexing
        tunnel: string[] ["Filter Size X", "Filter Size Y", "Tolerance %"] -> [w664]
        tunnel: string[] ["Kernel", "Kernel Size", "Divider"] -> [w663]
        tunnel: w649 -> [w657]
        tunnel: [w659] -> w648
        tunnel: string[] ["Sigma", "HThresh", "LThres", "Windows Size"] -> [w656]
        n197 = property class="Ctl"(reference=w658, error in=w657) -> (error out=w662:errorcluster, "Label.Text"=w655:string)  [unwired: 1 out]
        n198 = for {
          tunnel: w655 -> [w682]
          tunnel: w663 -> [w681] mode=indexing
          tunnel: w658 -> [w679]
          tunnel: w657 -> [w678]
          tunnel: [w677] -> w660
          n199 = Equal?(x=w682, y=w681) -> (x = y?=w680:bool)
          n200 = case shown="True" w680 {
            tunnel: w679 -> [_ w688]
            tunnel: w678 -> [w683 w686]
            tunnel: [w683 w685] -> w677
            frame False {
            }
            frame True {
              n201 = property class="Ctl"(reference=w688, error in=w686, "DisabledEnum"=T3."Disabled and Grayed Out" ("Disabled"), "Visible"=FALSE) -> (error out=w685:errorcluster)  [unwired: 1 out]
            }
          }
        }
        n202 = for {
          tunnel: w655 -> [w694]
          tunnel: w664 -> [w693] mode=indexing
          tunnel: w658 -> [w691]
          tunnel: w662 -> [w690]
          tunnel: [w689] -> w661
          n203 = Equal?(x=w694, y=w693) -> (x = y?=w692:bool)
          n204 = case shown="True" w692 {
            tunnel: w691 -> [_ w700]
            tunnel: w690 -> [w695 w698]
            tunnel: [w695 w697] -> w689
            frame False {
            }
            frame True {
              n205 = property class="Ctl"(reference=w700, error in=w698, "DisabledEnum"=T3."Disabled and Grayed Out" ("Disabled"), "Visible"=FALSE) -> (error out=w697:errorcluster)  [unwired: 1 out]
            }
          }
        }
        n206 = for {
          tunnel: w655 -> [w670]
          tunnel: w656 -> [w669] mode=indexing
          tunnel: w658 -> [w667]
          tunnel: w657 -> [w666]
          tunnel: [w665] -> _
          n207 = Equal?(x=w670, y=w669) -> (x = y?=w668:bool)
          n208 = case shown="True" w668 {
            tunnel: w667 -> [_ w676]
            tunnel: w666 -> [w671 w674]
            tunnel: [w671 w673] -> w665
            frame False {
            }
            frame True {
              n209 = property class="Ctl"(reference=w676, error in=w674, "DisabledEnum"=T3."Enabled" ("Disabled"), "Visible"=TRUE) -> (error out=w673:errorcluster)  [unwired: 1 out]
            }
          }
        }
        n210 = Merge Errors(w661, w660) -> (w659:errorcluster)
      }
    }
    frame "------------------------------------", Default {
    }
    frame "----------------------------------------" {
    }
  }
  "Error Out" <- w3
